vi "_Dequeue CSMQ.vi"(8 "Error in":errorcluster caption="Error in (no error)", 9 "Dequeue Timeout(0ms)":i32, 10 "State(s) in (\"\")":string, 11 "CSMQ in":T1) -> (0 "Error out":errorcluster, 2 "States Out":string, 3 "CSMQ out":T1)   [LabVIEW 2014, in "Communicable State Machine.lvlib"]
uses:
  Communicable State Machine.lvlib
  _CSMQ.ctl
  Typedef/_Cross JKISM State Data.ctl
  Typedef/_CSM_MSG_TYPE.ctl
  Typedef/_Cross JKISM State Response.ctl
  Typedef/_CSM_MODE.ctl
  Typedef/_CSM Status Change Event Data.ctl
  AdvanceAPI/CSM - Message Type.ctl
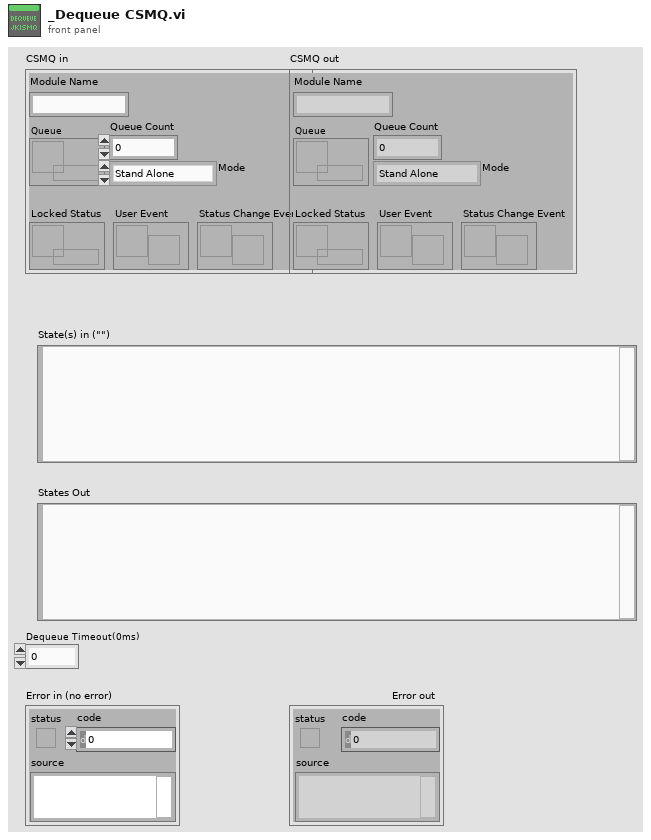
[diagram p1: front panel]
types:
  T1 = typedef "Communicable State Machine.lvlib/_CSMQ.ctl" = cluster{"Module Name":string, "Queue":refnum<queue>, "Locked Status":refnum<data-value>, "Mode":T2, "User Event":refnum<user-event>, "Queue Count":i32, "Status Change Event":refnum<user-event>}
  T2 = typedef "Communicable State Machine.lvlib/_CSM_MODE.ctl" = enum16{"Stand Alone", "JKISM", "Action Worker"}
  T3 = typedef "Communicable State Machine.lvlib/CSM - Message Type.ctl" = enum16{"Async", "Async without Reply", "Sync"}
  T4 = typedef "Communicable State Machine.lvlib/_Cross JKISM State Data.ctl" = cluster{"Msg Type":T5, "state":string, "args":string, "source":string, "RespQ":refnum<queue>, "Pre-State":string, "Arg-State":string, "Target":string}
  T5 = typedef "Communicable State Machine.lvlib/_CSM_MSG_TYPE.ctl" = enum16{"Sync Message(-@)", "Async Message(->)", "Async without Response(->|)", "Async Response", "Broadcast(-><status>)", "Broadcast(-><interrupt>)", "Request to Post Message", "Request to Post Message without Reply", "Request to Publish Status"}
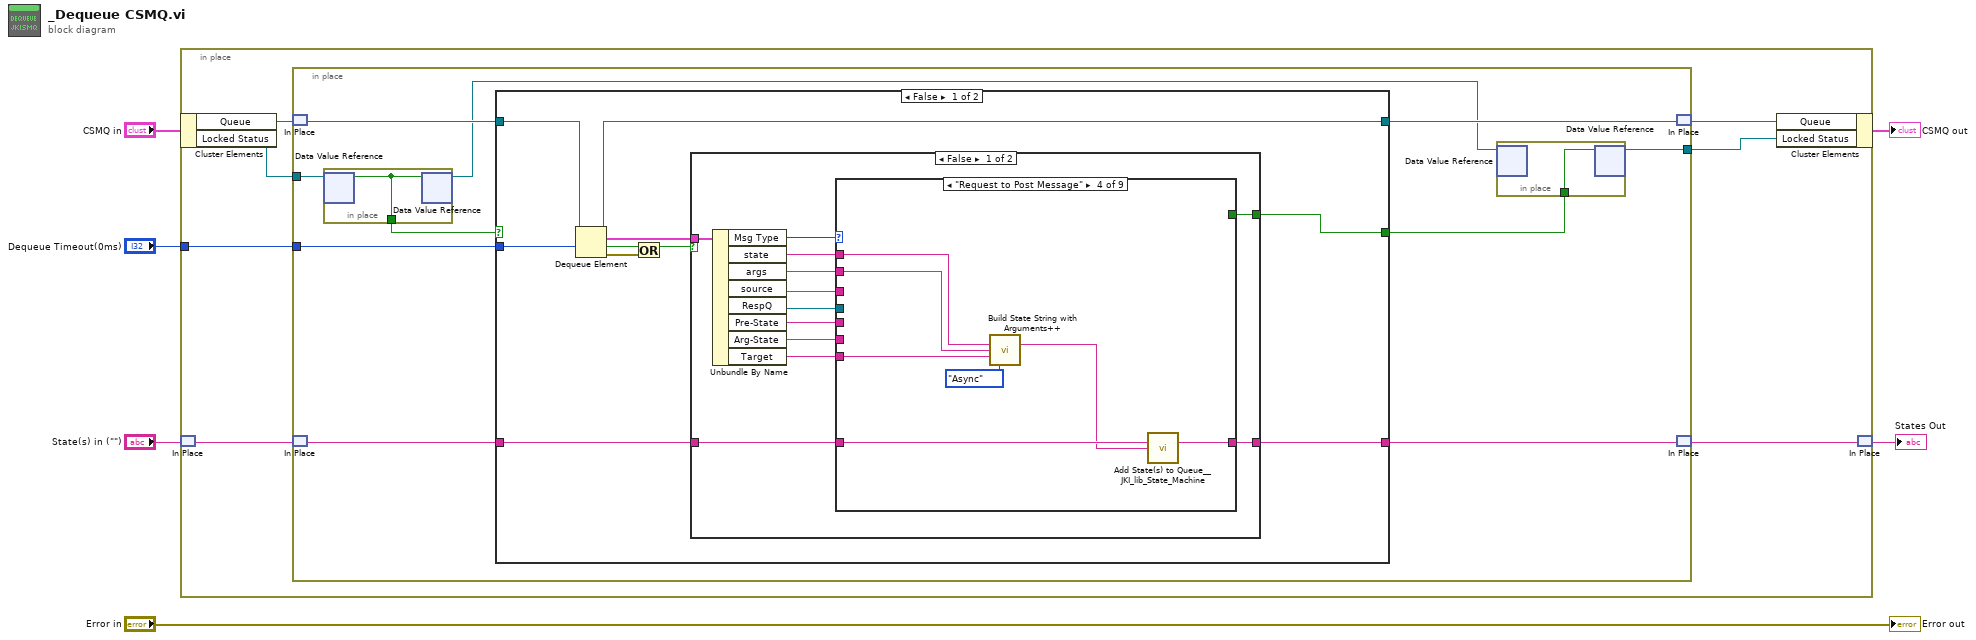
[diagram p0: block diagram]
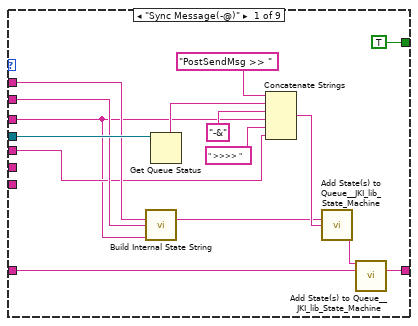
[diagram p2: hidden frame]
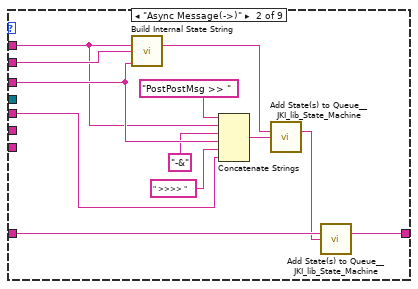
[diagram p3: hidden frame]
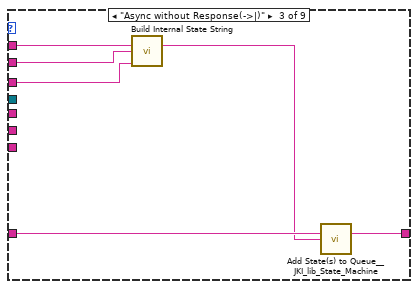
[diagram p4: hidden frame]
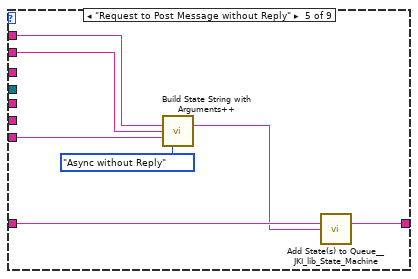
[diagram p5: hidden frame]
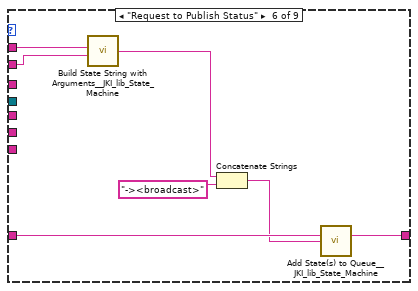
[diagram p6: hidden frame]
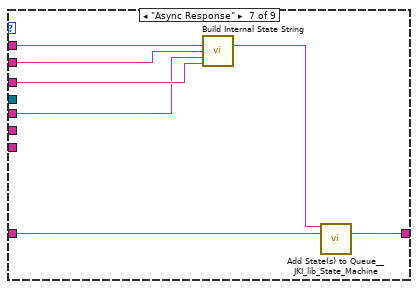
[diagram p7: hidden frame]
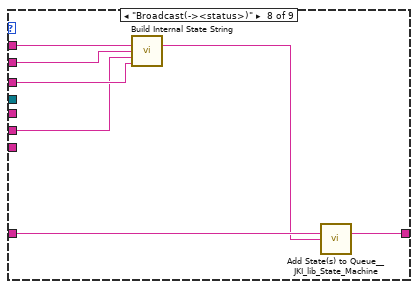
[diagram p8: hidden frame]
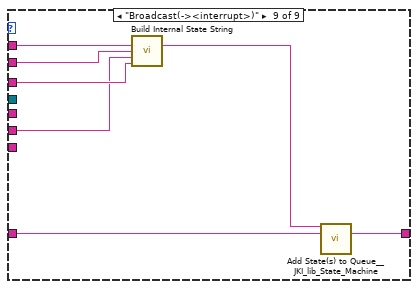
[diagram p9: hidden frame]
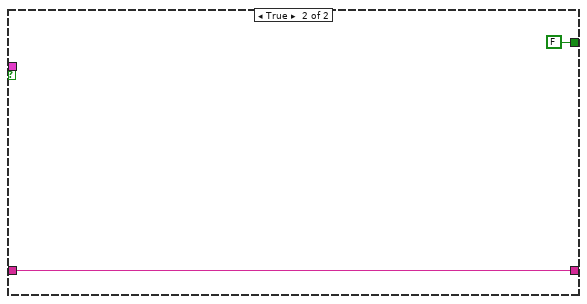
[diagram p10: hidden frame]
diagram:
  n1 = in-place "In Place Element Structure" {
    in-place-border: "Dequeue Timeout(0ms)" -> [w11]
    n2 = in-place-cluster #1("CSMQ in") -> ("Queue"=w13:refnum<queue>, "Locked Status"=w8:refnum<data-value>)
    n3 = in-place-match #2("State(s) in (\"\")") -> (w10:string)
    n4 = in-place {
      in-place-border: w11 -> [w21]
      in-place-border: w8 -> [w18]
      in-place-border: [w15] -> w7
      n5 = in-place-match #3(w13) -> (w22:refnum<queue>)
      n6 = in-place-match #4(w10) -> (w20:string)
      n7 = in-place {
        in-place-border: [w25] -> w17
        n8 = in-place-dvr #5(w18) -> (w25:bool)  [unwired: 1 out]
        n9 = in-place-dvr #5(w25) -> (w16:refnum<data-value>)  [unwired: 1 out]
      }
      n10 = case shown="False" w17 {
        selector: w17 -> [_ w125]
        tunnel: [w34 w127] -> w23
        tunnel: w22 -> [w35 w127]
        tunnel: w21 -> [w33 _]
        tunnel: w20 -> [w31 w126]
        tunnel: [w30 w126] -> w19
        tunnel: [w29 w125] -> w14
        frame False {
          n11 = Dequeue Element(queue=w35, timeout in ms (-1)=w33) -> (queue out=w34:refnum<queue>, element=w32:T4, timed out?=w27:bool, error out=w26:errorcluster)  [unwired: 1 in]
          n12 = Or(x=w27, y=w26) -> (x .or. y?=w28:bool)
          n13 = case shown="False" w28 {
            tunnel: w31 -> [w47 w124]
            tunnel: [w46 w124] -> w30
            tunnel: w32 -> [w41 _]
            tunnel: [w40 FALSE] -> w29
            frame False {
              n14 = Unbundle By Name(w41) -> ("Msg Type"=w37:T5, "state"=w44:string, "args"=w43:string, "source"=w42:string, "RespQ"=w45:refnum<queue>, "Pre-State"=w39:string, "Arg-State"=w38:string, "Target"=w36:string)
              n15 = case shown="\"Request to Post Message\"" w37 {
                tunnel: w47 -> [w62 w74 w80 w87 w94 w101 w108 w115 w122]
                tunnel: [w61 w73 w79 w86 w93 w100 w107 w114 w121] -> w46
                tunnel: w45 -> [w60 _ _ _ _ _ _ _ _]
                tunnel: w44 -> [w55 w70 w76 w85 w92 w97 w104 w111 w118]
                tunnel: w43 -> [w54 w72 w78 w84 w91 w96 w106 w113 w120]
                tunnel: w42 -> [w48 w71 w77 _ _ _ w105 w112 w119]
                tunnel: [TRUE _ _ _ _ _ _ _ _] -> w40
                tunnel: w39 -> [w49 w69 _ _ _ _ w103 _ _]
                tunnel: w38 -> [_ _ _ _ _ _ _ w110 w117]
                tunnel: w36 -> [_ _ _ w83 w90 _ _ _ _]
                frame "Sync Message(-@)" {
                  n16 = call "Build Internal State String.vi"("State"=w55, "Arguments (\"\")"=w54, "Source (\"\")"=w48) -> ("State with Arguments"=w56:string)  [unwired: 12 in]
                  n17 = Get Queue Status(queue=w60) -> (queue name=w53:string)  [unwired: 2 in, 7 out]
                  n18 = Concatenate Strings("PostSendMsg >> " ("State(s) at Back (\"\")"), w53, "-&" ("string"), w48, " >>>> " ("string"), w49) -> (w57:string)
                  n19 = call <vilib>:"Add State(s) to Queue__JKI_lib_State_Machine.vi"("State(s) in (\"\")"=w56, "State(s) at Back (\"\")"=w57) -> ("States Out"=w59:string)  [unwired: 13 in]
                  n20 = call <vilib>:"Add State(s) to Queue__JKI_lib_State_Machine.vi"("State(s) in Front (\"\")"=w59, "State(s) in (\"\")"=w62) -> ("States Out"=w61:string)  [unwired: 13 in]
                }
                frame "Async Message(->)" {
                  n21 = call "Build Internal State String.vi"("State"=w70, "Arguments (\"\")"=w72, "Source (\"\")"=w71) -> ("State with Arguments"=w65:string)  [unwired: 12 in]
                  n22 = Concatenate Strings("PostPostMsg >> " ("State(s) at Back (\"\")"), w70, "-&" ("string"), w71, " >>>> " ("string"), w69) -> (w64:string)
                  n23 = call <vilib>:"Add State(s) to Queue__JKI_lib_State_Machine.vi"("State(s) in (\"\")"=w65, "State(s) at Back (\"\")"=w64) -> ("States Out"=w68:string)  [unwired: 13 in]
                  n24 = call <vilib>:"Add State(s) to Queue__JKI_lib_State_Machine.vi"("State(s) in (\"\")"=w74, "State(s) at Back (\"\")"=w68) -> ("States Out"=w73:string)  [unwired: 13 in]
                }
                frame "Async without Response(->|)" {
                  n25 = call "Build Internal State String.vi"("State"=w76, "Arguments (\"\")"=w78, "Source (\"\")"=w77) -> ("State with Arguments"=w75:string)  [unwired: 12 in]
                  n26 = call <vilib>:"Add State(s) to Queue__JKI_lib_State_Machine.vi"("State(s) in (\"\")"=w80, "State(s) at Back (\"\")"=w75) -> ("States Out"=w79:string)  [unwired: 13 in]
                }
                frame "Request to Post Message" {
                  n27 = call "Build State String with Arguments++.vi"("State"=w85, "Arguments (\"\")"=w84, "Target Module (\"\")"=w83, "Type"=CSM_-_Message_Type."Async") -> ("State with Arguments"=w82:string)  [unwired: 11 in]
                  n28 = call <vilib>:"Add State(s) to Queue__JKI_lib_State_Machine.vi"("State(s) in (\"\")"=w87, "State(s) at Back (\"\")"=w82) -> ("States Out"=w86:string)  [unwired: 13 in]
                }
                frame "Request to Post Message without Reply" {
                  n29 = call "Build State String with Arguments++.vi"("State"=w92, "Arguments (\"\")"=w91, "Target Module (\"\")"=w90, "Type"=CSM_-_Message_Type."Async without Reply") -> ("State with Arguments"=w89:string)  [unwired: 11 in]
                  n30 = call <vilib>:"Add State(s) to Queue__JKI_lib_State_Machine.vi"("State(s) in (\"\")"=w94, "State(s) at Back (\"\")"=w89) -> ("States Out"=w93:string)  [unwired: 13 in]
                }
                frame "Request to Publish Status" {
                  n31 = call <vilib>:"Build State String with Arguments__JKI_lib_State_Machine.vi"("Arguments (\"\")"=w96, "State"=w97) -> ("State with Arguments"=w95:string)  [unwired: 4 in]
                  n32 = Concatenate Strings(w95, "-><broadcast>" ("string")) -> (w98:string)
                  n33 = call <vilib>:"Add State(s) to Queue__JKI_lib_State_Machine.vi"("State(s) in (\"\")"=w101, "State(s) at Back (\"\")"=w98) -> ("States Out"=w100:string)  [unwired: 13 in]
                }
                frame "Async Response" {
                  n34 = call "Build Internal State String.vi"("State"=w104, "Arguments (\"\")"=w106, "Arg-State (\"\")"=w103, "Source (\"\")"=w105) -> ("State with Arguments"=w102:string)  [unwired: 11 in]
                  n35 = call <vilib>:"Add State(s) to Queue__JKI_lib_State_Machine.vi"("State(s) in Front (\"\")"=w102, "State(s) in (\"\")"=w108) -> ("States Out"=w107:string)  [unwired: 13 in]
                }
                frame "Broadcast(-><status>)" {
                  n36 = call "Build Internal State String.vi"("State"=w111, "Arguments (\"\")"=w113, "Arg-State (\"\")"=w110, "Source (\"\")"=w112) -> ("State with Arguments"=w109:string)  [unwired: 11 in]
                  n37 = call <vilib>:"Add State(s) to Queue__JKI_lib_State_Machine.vi"("State(s) in (\"\")"=w115, "State(s) at Back (\"\")"=w109) -> ("States Out"=w114:string)  [unwired: 13 in]
                }
                frame "Broadcast(-><interrupt>)" {
                  n38 = call "Build Internal State String.vi"("State"=w118, "Arguments (\"\")"=w120, "Arg-State (\"\")"=w117, "Source (\"\")"=w119) -> ("State with Arguments"=w116:string)  [unwired: 11 in]
                  n39 = call <vilib>:"Add State(s) to Queue__JKI_lib_State_Machine.vi"("State(s) in Front (\"\")"=w116, "State(s) in (\"\")"=w122) -> ("States Out"=w121:string)  [unwired: 13 in]
                }
              }
            }
            frame True {
            }
          }
        }
        frame True {
        }
      }
      n40 = in-place {
        in-place-border: w14 -> [w24]
        n41 = in-place-dvr #6(w16) -> ()  [unwired: 2 out]
        n42 = in-place-dvr #6(w24) -> (w15:refnum<data-value>)  [unwired: 1 out]
      }
      n43 = in-place-match #3(w23) -> (w12:refnum<queue>)
      n44 = in-place-match #4(w19) -> (w9:string)
    }
    n45 = in-place-cluster #1("Queue"=w12, "Locked Status"=w7) -> (→"CSMQ out":T1)
    n46 = in-place-match #2(w9) -> (→"States Out":string)
  }
  "Error out" <- "Error in"
